vi "uittesten_PID (SubVI).vi"() -> ()   [LabVIEW 2019]
uses:
  <vilib>/addons/control/pid/pid.llb/PID (DBL).vi
  <vilib>/addons/control/pid/NI_PID_pid.lvlib
panel:
  out "output":dbl format="%.2f"
  out "Gauge":cluster{dbl, dbl}(knob)={0.0, 3.638763258839615} scale=0.0..10.0
  in  "Slide":dbl(slide) scale=0.0..10.0
  in  "PID gains":T1={"proportional gain (Kc)"=1.0, "integral time (Ti, min)"=0.01, "derivative time (Td, min)"=0.0} {"derivative time (Td, min)" format="%.3f"; "integral time (Ti, min)" format="%.3f"; "proportional gain (Kc)" format="%.3f"}
  in  "output range":cluster{"output high":dbl, "output low":dbl}={"output high"=100.0, "output low"=-100.0} {"output low" format="%.2f"; "output high" format="%.2f"}
  in  "stop":bool
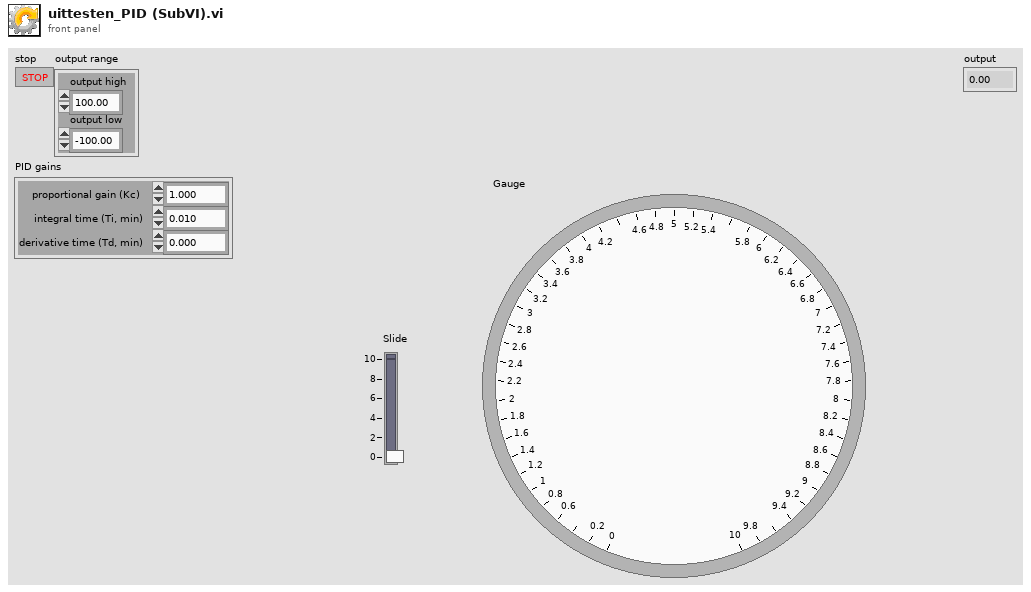
[diagram p1: front panel]
types:
  T1 = cluster{"proportional gain (Kc)":dbl, "integral time (Ti, min)":dbl, "derivative time (Td, min)":dbl}
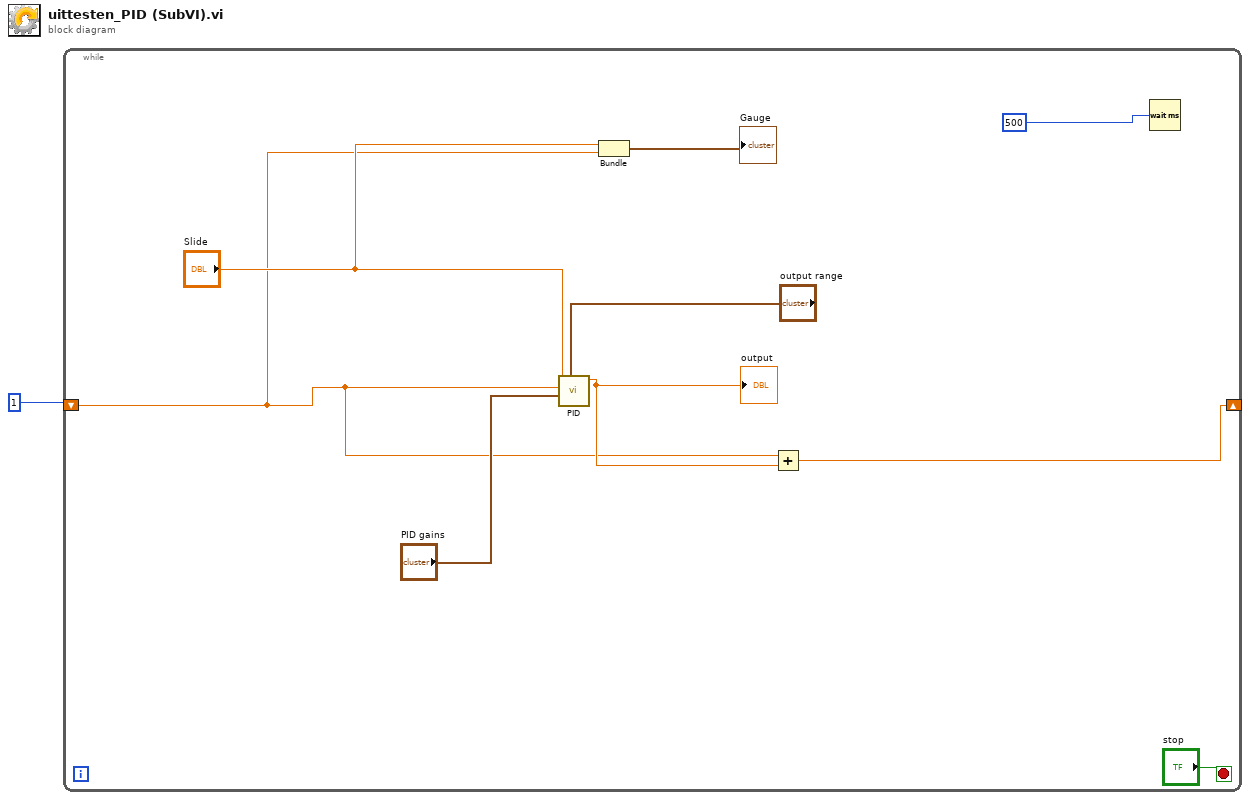
[diagram p0: block diagram]
diagram:
  n1 = while {
    shift-right: [w7] -> _
    shift-left: 1 -> [w3]
    stop <- "stop" stop-if-true
    n2 = call-poly <vilib>:"PID.vi"("output range"="output range", "PID gains"="PID gains", "process variable"=w3, "setpoint"="Slide") -> ("output"=w5:dbl)  [unwired: 6 in, 1 out]
    "output" <- w5
    n3 = Bundle("Slide"="Slide", w3) -> (→"Gauge":cluster{"Slide":dbl, dbl})  [unwired: 1 in]
    n4 = Add(x=w3, y=w5) -> (x+y=w7:dbl)
    n5 = Wait (ms)(milliseconds to wait=500) -> ()  [unwired: 1 out]
  }
